vi "c_ctre_phoenix6_platform_replay_get_double_array.vi"(0 "String 2":string, 1 "Numeric 3":u32, 2 "Numeric 5":dbl, 3 "Numeric 7":u8, 4 "Numeric 9":dbl) -> (20 "Numeric":i32, 21 "String":string, 22 "Numeric 2":u32, 23 "Numeric 4":dbl, 24 "Numeric 6":u8, 25 "Numeric 8":dbl)   [LabVIEW 2023]
uses:
  <vilib>/Rock Robotics/WPI/ThirdParty/Phoenix-LabVIEW/Controls/DriverLib.ctl
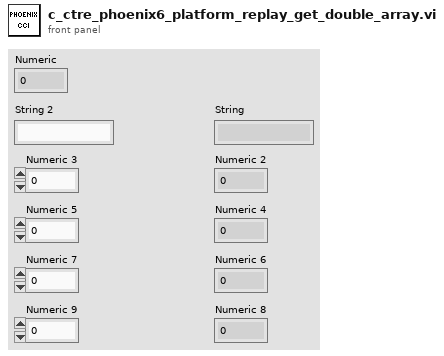
[diagram p1: front panel]
types:
  T1 = typedef "DriverLib.ctl" = path
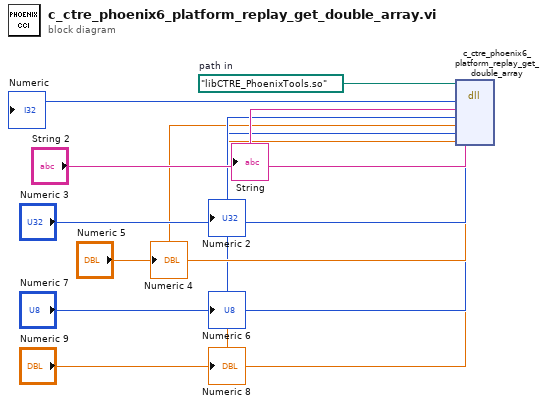
[diagram p0: block diagram]
diagram:
  w12 = T1 path "libCTRE_PhoenixTools.so"  # path in
  n1 = dll-call lib="?" fn="c_ctre_phoenix6_platform_replay_get_double_array"(path in=w12, "String 2", "Numeric 3", "Numeric 5", "Numeric 7", "Numeric 9") -> (→"Numeric":i32, →"String":string, →"Numeric 2":u64, →"Numeric 4":dbl, →"Numeric 6":u8, →"Numeric 8":dbl)  [unwired: 2 in, 2 out]
